vi "Microphone Test.vi"(5 "Test Configuration":T2, 8 "error in (no error)":errorcluster, 10 "Mic Command":u8, 11 "Session Handle in":T1) -> (0 "error out":errorcluster, 1 "ADC":dbl, 2 "Success?":bool, 3 "Session Handle out":T1)   [LabVIEW 2015, in "PAS.lvclass"]
uses:
  PAS.lvclass
  Typedefs/Session Handle.ctl
  Tests/Controls/Test Configuration.ctl
  Tests/Controls/Vacuum Test.ctl
  Tests/Controls/Test Timing.ctl
  Tests/Controls/Vaccum Thresholds.ctl
  Tests/Controls/Helium Test.ctl
  Tests/Controls/Helium Thresholds.ctl
  Tests/Controls/Functional Test.ctl
  Typedefs/Emitter Power.ctl
  Typedefs/Valves.ctl
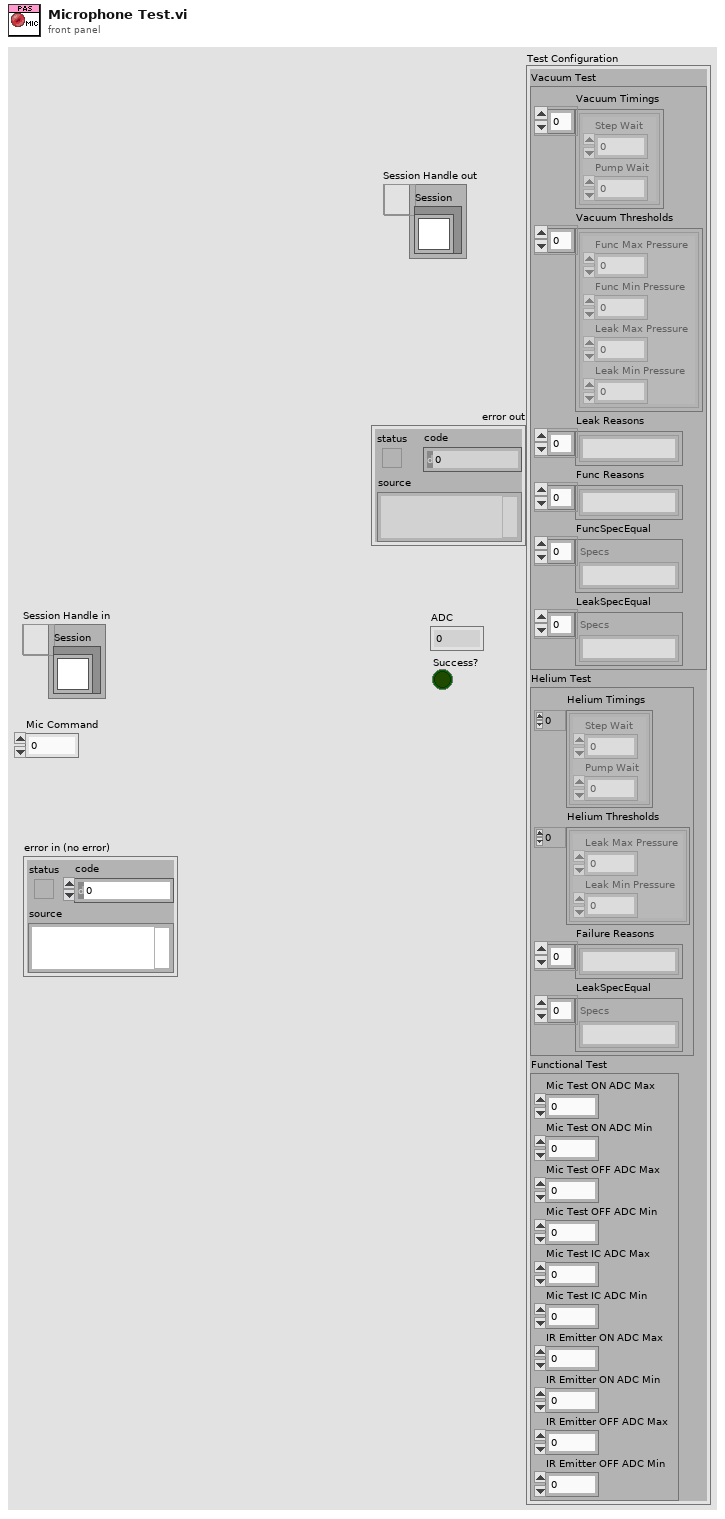
[diagram p1: front panel]
types:
  T1 = typedef "PAS.lvclass/Session Handle.ctl" = refnum<data-value>
  T2 = typedef "Test Configuration.ctl" = cluster{"Vacuum Test":T3, "Helium Test":T6, "Functional Test":T8}
  T3 = typedef "Vacuum Test.ctl" = cluster{"Vacuum Timings":T4[], "Vacuum Thresholds":T5[], "Leak Reasons":string[], "Func Reasons":string[], "FuncSpecEqual":string[], "LeakSpecEqual":string[]}
  T4 = typedef "Test Timing.ctl" = cluster{"Step Wait":dbl, "Pump Wait":dbl}
  T5 = typedef "Vaccum Thresholds.ctl" = cluster{"Func Max Pressure":dbl, "Func Min Pressure":dbl, "Leak Max Pressure":dbl, "Leak Min Pressure":dbl}
  T6 = typedef "Helium Test.ctl" = cluster{"Helium Timings":T4[], "Helium Thresholds":T7[], "Failure Reasons":string[], "LeakSpecEqual":string[]}
  T7 = typedef "Helium Thresholds.ctl" = cluster{"Leak Max Pressure":dbl, "Leak Min Pressure":dbl}
  T8 = typedef "Functional Test.ctl" = cluster{"Mic Test ON ADC Max":dbl, "Mic Test ON ADC Min":dbl, "Mic Test OFF ADC Max":dbl, "Mic Test OFF ADC Min":dbl, "Mic Test IC ADC Max":dbl, "Mic Test IC ADC Min":dbl, "IR Emitter ON ADC Max":dbl, "IR Emitter ON ADC Min":dbl, "IR Emitter OFF ADC Max":dbl, "IR Emitter OFF ADC Min":dbl}
  T9 = typedef "PAS.lvclass/Valves.ctl" = u16
  T10 = typedef "PAS.lvclass/Emitter Power.ctl" = u16
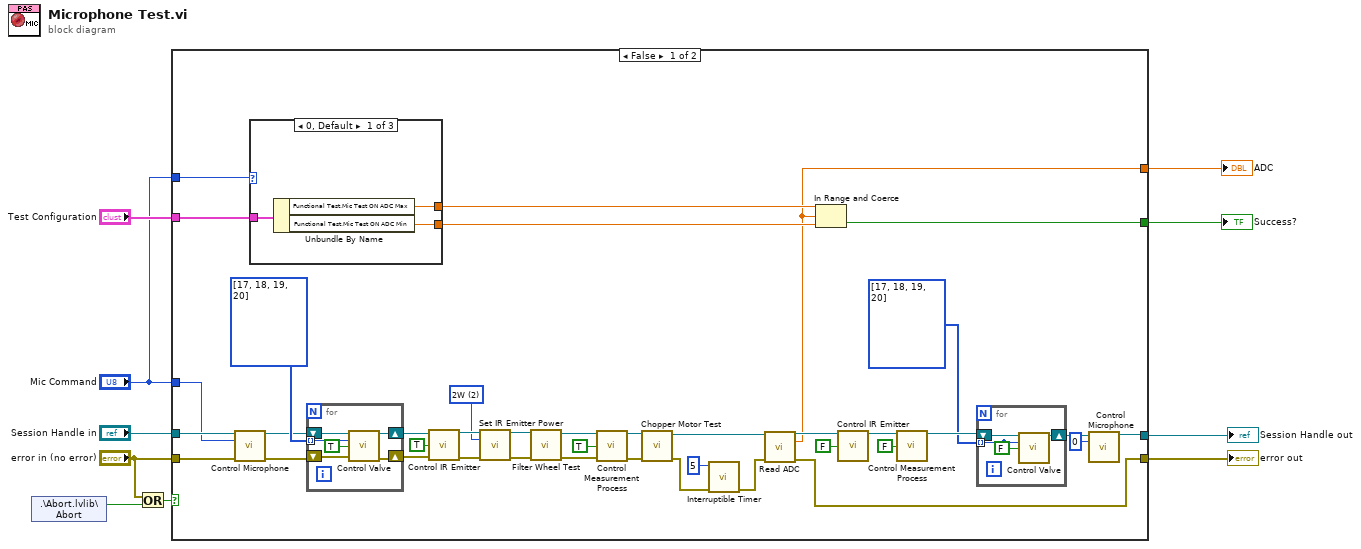
[diagram p0: block diagram]
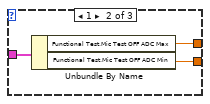
[diagram p2: hidden frame]
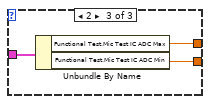
[diagram p3: hidden frame]
diagram:
  n1 = shared-variable ".\\Abort.lvlib\\Abort"() -> (w4:bool)  [unwired: 1 in, 1 out]
  n2 = Or(x="error in (no error)", y=w4) -> (x .or. y?=w6:bool)
  n3 = case shown="False" w6 {
    tunnel: "Test Configuration" -> [w39 _]
    tunnel: "Session Handle in" -> [w36 w70]
    tunnel: "error in (no error)" -> [w35 w69]
    tunnel: [w12 w70] -> w8
    tunnel: [w20 w69] -> w7
    tunnel: [w17 _] -> w3
    tunnel: [w16 _] -> w2
    tunnel: "Mic Command" -> [w15 _]
    tunnel: "Mic Command" -> [w14 _]
    frame False {
      w21 = T9[] [17, 18, 19, 20] items=["PV1"=17, "PV2"=18, "PV3"=19, "PV4"=20]
      w43 = T10 2 items=["2W"=2, "3W"=3, "4W"=4, "5W"=5] ("Emitter Power")
      w49 = T9[] [17, 18, 19, 20] items=["PV1"=17, "PV2"=18, "PV3"=19, "PV4"=20]
      n4 = call "Control Microphone.vi"("Session Handle in"=w36, "Command"=w15, "error in (no error)"=w35) -> ("Session Handle out"=w38:T1, "error out"=w37:errorcluster)  [unwired: 9 in, 2 out]
      n5 = case shown="0, Default" w14 {
        tunnel: w39 -> [w52 w55 w58]
        tunnel: [w51 w54 w57] -> w19
        tunnel: [w50 w53 w56] -> w18
        frame 0, Default {
          n6 = Unbundle By Name(w52) -> ("Functional Test.Mic Test ON ADC Max"=w51:dbl, "Functional Test.Mic Test ON ADC Min"=w50:dbl)
        }
        frame 1 {
          n7 = Unbundle By Name(w55) -> ("Functional Test.Mic Test OFF ADC Max"=w54:dbl, "Functional Test.Mic Test OFF ADC Min"=w53:dbl)
        }
        frame 2 {
          n8 = Unbundle By Name(w58) -> ("Functional Test.Mic Test IC ADC Max"=w57:dbl, "Functional Test.Mic Test IC ADC Min"=w56:dbl)
        }
      }
      n9 = for {
        shift-right: [w64] -> w48
        shift-left: w38 -> [w68]
        shift-right: [w65] -> w47
        shift-left: w37 -> [w66]
        tunnel: w49 -> [w67] mode=indexing
        n10 = call "Control Valve.vi"("Session Handle in"=w68, "Valves"=w67, "Energize?"=TRUE, "error in (no error)"=w66) -> ("Session Handle out"=w64:T1, "error out"=w65:errorcluster)  [unwired: 8 in, 2 out]
      }
      n11 = call "Control IR Emitter.vi"("Session Handle in"=w48, "Start?"=TRUE, "error in (no error)"=w47) -> ("Session Handle out"=w45:T1, "error out"=w44:errorcluster)  [unwired: 9 in, 2 out]
      n12 = call "Set IR Emitter Power.vi"("Session Handle in"=w45, "Emitter Power"=w43, "error in (no error)"=w44) -> ("Session Handle out"=w34:T1, "error out"=w33:errorcluster)  [unwired: 10 in, 1 out]
      n13 = call "Filter Wheel Test.vi"("error in (no error)"=w33, "Session Handle in"=w34) -> ("error out"=w31:errorcluster, "Session Handle out"=w32:T1)  [unwired: 7 in, 1 out]
      n14 = call "Control Measurement Process.vi"("Session Handle in"=w32, "Start?"=TRUE, "error in (no error)"=w31) -> ("Session Handle out"=w30:T1, "error out"=w29:errorcluster)  [unwired: 9 in, 2 out]
      n15 = call "Chopper Motor Test.vi"("error in (no error)"=w29, "Session Handle in"=w30) -> ("error out"=w28:errorcluster, "Session Handle out"=w25:T1)  [unwired: 7 in, 1 out]
      n16 = call "Interruptible Timer.vi"("error in (no error)"=w28, "Wait (s)"=5) -> ("error out"=w26:errorcluster)  [unwired: 7 in, 2 out]
      n17 = call "Read ADC.vi"("Session Handle in"=w25, "error in (no error)"=w26) -> ("Session Handle out"=w40:T1, "ADC"=w17:dbl, "error out"=w20:errorcluster)  [unwired: 10 in, 1 out]
      n18 = In Range and Coerce(upper limit=w19, x=w17, lower limit=w18) -> (In Range?=w16:bool)  [unwired: 1 out]
      n19 = call "Control IR Emitter.vi"("Session Handle in"=w40, "Start?"=FALSE) -> ("Session Handle out"=w24:T1)  [unwired: 10 in, 3 out]
      n20 = call "Control Measurement Process.vi"("Session Handle in"=w24, "Start?"=FALSE) -> ("Session Handle out"=w22:T1)  [unwired: 10 in, 3 out]
      n21 = for {
        shift-right: [w61] -> w13
        shift-left: w22 -> [w62]
        tunnel: [w59] -> _ mode=indexing
        tunnel: w21 -> [w59] mode=indexing
        n22 = call "Control Valve.vi"("Session Handle in"=w62, "Valves"=w59, "Energize?"=FALSE) -> ("Session Handle out"=w61:T1)  [unwired: 9 in, 3 out]
      }
      n23 = call "Control Microphone.vi"("Session Handle in"=w13, "Command"=u8 0) -> ("Session Handle out"=w12:T1)  [unwired: 10 in, 3 out]
    }
    frame True {
    }
  }
  "error out" <- w7
  "Session Handle out" <- w8
  "ADC" <- w3
  "Success?" <- w2
